vi "main program.vi"() -> ()   [LabVIEW 2015]
uses:
  <vilib>/rvi/interface/nirviReadWriteControl/nirviReadWriteControl.xnode
  <vilib>/rvi/interface/nirviMethod/nirviMethod.xnode
  <vilib>/rvi/interface/nirviCloseFPGA/nirviCloseFPGA.xnode
  <vilib>/FPGAPlugInAG/Dynamic/niLvFpga_Run_Dynamic.vi
  <vilib>/rvi/interface/Simulation/niFpgaSimulationCallBeginRW.vi
  <vilib>/rvi/errors/niLvFpgaAdjustHostInterfaceError.vi
  <vilib>/Platform/TimedLoop/XDataNode/XDataNode.xnode
  <vilib>/Platform/TimedLoop/XDataNode/nitl_modes.ctl
  <vilib>/Platform/TimedLoop/XDataNode/XDNodeRunTimeDep.lvlib
  <vilib>/Platform/TimedLoop/XDataNode/wakeup.ctl
  <vilib>/Platform/TimedLoop/XDataNode/timing_clust.ctl
  <vilib>/FPGAPlugInAG/Dynamic/niLvFpga_Close_Dynamic.vi
  <vilib>/vision/driver/NI_Vision_Acquisition_Software.lvlib
  <resource>/objmgr/imaqdx.rc
  <vilib>/addons/control/pid/NI_PID_pid.lvlib
  <vilib>/addons/control/pid/pid.llb/PID (DBL).vi
  <vilib>/addons/Fuzzy Logic/NI_Fuzzy_Logic_API.lvlib
  <vilib>/addons/Fuzzy Logic/FL Fuzzy Controller (MIMO).vi
  <vilib>/rvi/interface/nirviOpenFPGA/nirviOpenFPGA.xnode
  NiFpgaLv.dll
  <vilib>/Utility/error.llb/Error Cluster From Error Code.vi
  <vilib>/rvi/Arithmetic/AddSubMult/XNode/nirviSatArithmetic.xnode
  FPGA Bitfiles/FPGAv2_FPGATarget2_Assemble3_74ibksKrDUk.lvbitx
  Assemble.vi
  <vilib>/FPGAPlugInAG/myRIO-1900/niLvFpga_Open_myRIO-1900.vi
  <vilib>/rvi/interface/common/dynamic/niFpgaDynamicAddResources.vi
  <vilib>/userdefined/High Color/IMAQdx.ctl
panel:
  out "Battery percentage":dbl(slide) scale=0.0..100.0
  in  "file path":path=path "c:/captue.jpg"
  out "Distance":dbl
  in  "Capture pict.":bool
  out "video modes":string
  in  "video mode":u32=20
  out "?":T1(plugin-control)
  in  "webcam":T2="cam0"
  out "k.kanan":dbl
  out "k.kiri":dbl
  out "x-y 2":dbl
  out "x+y 2":dbl
  out "percp. 2":dbl
  out "w 2":dbl
  out "percp.":dbl
  out "w":dbl
  out "Velo":i32
  out "Acce":i32
  in  "interval 2":u32=1000
  out "Vel":i32
  out "Acc":i32
  in  "interval":u32=1000
  out "x-y":dbl
  out "x+y":dbl
  out "b":dbl
  out "a":dbl
  out "Velocity (Counts/Interval) 4":i32
  out "Velocity (Counts/Interval) 3":i32
  out "Velocity (Counts/Interval) 2":i32
  out "Velocity (Counts/Interval)":i32
  out "Acceleration (rps/s) 4":dbl
  out "Acceleration (rps/s) 3":dbl
  out "Acceleration (rps/s) 2":dbl
  out "Acceleration (rps/s)":dbl
  out "frame rate [fps]":dbl
  out "STOP Indicator":bool
  in  "Run/Stop":bool
  out "RC ch3":u32
  out "heading error":dbl
  out "target bearing":dbl
  out "target distance":dbl
  in  "y target":dbl
  in  "x target":dbl
  out "voltage":dbl
  out "var.RTH":dbl
  out "kec.kanan":dbl
  out "kec.kiri":dbl
  out "kecp.kanan":dbl
  out "kecp.kiri":dbl
  out "var.auto":dbl
  in  "Mode":bool
  in  "RTH":bool
  out "relay 4":bool
  out "relay 3":bool
  out "relay 2":bool
  out "relay1":bool
  out "bocor 2":bool
  out "Water_LVL2":dbl
  out "Water_LVL1":dbl
  out "bocor 1":bool
  out "Arus 4":dbl
  out "Arus 3":dbl
  out "Arus1":dbl
  out "Arus2":dbl
  out "En 8":bool
  out "En 7":bool
  out "En 6":bool
  out "En 5":bool
  out "En 4":bool
  out "En 3":bool
  out "En 2":bool
  out "En 1":bool
  out "Rpm 4":dbl
  out "Rpm 3":dbl
  out "Rpm 2":dbl
  out "Rpm 1":dbl
  out "To":dbl
  out "var. manual":dbl
  out "enc 4":i32
  out "enc 3":i32
  out "enc 2":i32
  out "enc 1":i32
  out "Time On4":dbl format="%.2f"
  out "Time On3":dbl format="%.2f"
  out "Time On2":dbl
  out "y position":dbl
  out "x position":dbl
  out "angle":dbl
  out "Toff":dbl
  out "Time On1":dbl
  out "ultrasonik4":sgl
  out "ultrasonik3":sgl
  out "ultrasonik2":sgl
  out "ultrasonik1":sgl
  out "RC ch2":u32
  out "RC ch1":u32
  out "US 4":u32
  out "US3":u32
  out "US2":u32
  out "US1":u32
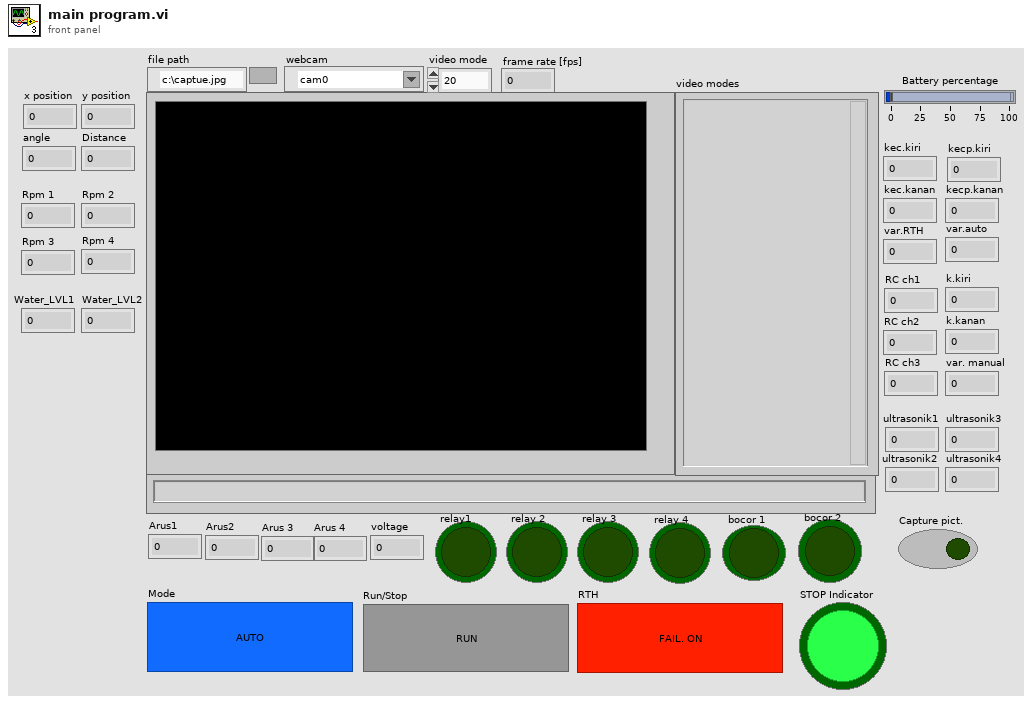
[diagram p1: front panel]
types:
  T1 = typedef "IMAQ Image.ctl" = refnum<image>
  T2 = typedef "IMAQdx.ctl" = refnum<k21>
  T3 = cluster{"Video Mode":u32, "Video Mode Name":string}[]
  T4 = typedef "XDNodeRunTimeDep.lvlib/timing_clust.ctl" = cluster{"Expected End [f-1]":u64, "Actual End [f-1]":u64, "Finished Late? [f-1]":bool, "Expected End [i-1]":u64, "Actual End [i-1]":u64, "Finished Late? [i-1]":bool, "Expected Start [i]":u64, "Actual Start [i]":u64, "Expected Start [f]":u64, "Actual Start [f]":u64, "Source Name":string, "Structure Name":string, "Period":i64, "Deadline":i64, "Offset":i64, "Start":i64, "Priority":i32, "Timeout":i32, "Mode":T5, "Wakeup Reason":T6, "Error":errorcluster, "Source Type":string, "Secondary Source Type":string, "Global End Time":u64, "Global Start Time":u64, "Frame Duration":u64, "Iteration Duration":u64, "Assigned CPU":i32, "I/O Scan Engine Mode":u32}
  T5 = typedef "XDNodeRunTimeDep.lvlib/nitl_modes.ctl" = enum32{"No Change", "Process missed periods, maintain original phase", "Discard missed periods, maintain original phase", "Process missed periods, ignore original phase", "Discard missed periods, ignore original phase"}
  T6 = typedef "XDNodeRunTimeDep.lvlib/wakeup.ctl" = enum32{"Normal", "Aborted", "Asynchronous wakeup", "Timing source error", "Timed loop error", "Timeout"}
  T7 = cluster{"proportional gain (Kc)":dbl, "integral time (Ti, min)":dbl, "derivative time (Td, min)":dbl}
  T8 = typedef "NI_Fuzzy_Logic_API.lvlib/FL System.ctl" = cluster{"input variables":T9[], "output variables":T9[], "rules":T12[], "defuzzification method":T18, "description":string, "user MF interpolating polynomials":T19[]}
  T9 = typedef "NI_Fuzzy_Logic_API.lvlib/FL Variable.ctl" = cluster{"name":string, "range":dbl[], "MFs":T10[]}
  T10 = typedef "NI_Fuzzy_Logic_API.lvlib/FL Membership Function.ctl" = cluster{"name":string, "shape":T11, "points":dbl[], "color":u32, "user-defined shape index":i32}
  T11 = typedef "NI_Fuzzy_Logic_API.lvlib/FL Membership Function Shape.ctl" = u16
  T12 = typedef "NI_Fuzzy_Logic_API.lvlib/FL Rule.ctl" = cluster{"antecedents":T13[], "antecedent connective":T15, "consequents":T16[], "consequent implication":T17, "degree of support":dbl}
  T13 = typedef "NI_Fuzzy_Logic_API.lvlib/FL Antecedent.ctl" = cluster{"Var Index":i32, "MF Index":i32, "Cond":T14}
  T14 = typedef "NI_Fuzzy_Logic_API.lvlib/FL Modifier.ctl" = u16
  T15 = typedef "NI_Fuzzy_Logic_API.lvlib/FL Antecedent Connective.ctl" = u16
  T16 = typedef "NI_Fuzzy_Logic_API.lvlib/FL Consequent.ctl" = cluster{"Var Index":i32, "MF Index":i32, "Cond":T14}
  T17 = typedef "NI_Fuzzy_Logic_API.lvlib/FL Consequent Implication.ctl" = u16
  T18 = typedef "NI_Fuzzy_Logic_API.lvlib/FL Defuzzification.ctl" = u16
  T19 = typedef "NI_Fuzzy_Logic_API.lvlib/FL Interpolating polynomials.ctl" = cluster{"X":dbl[], "Y":dbl[], "Y(x) coeff":dbl[][], "X(y) coeff":dbl[][], "Area(y) coeff":dbl[][], "coa_x(y) coeff":dbl[][]}
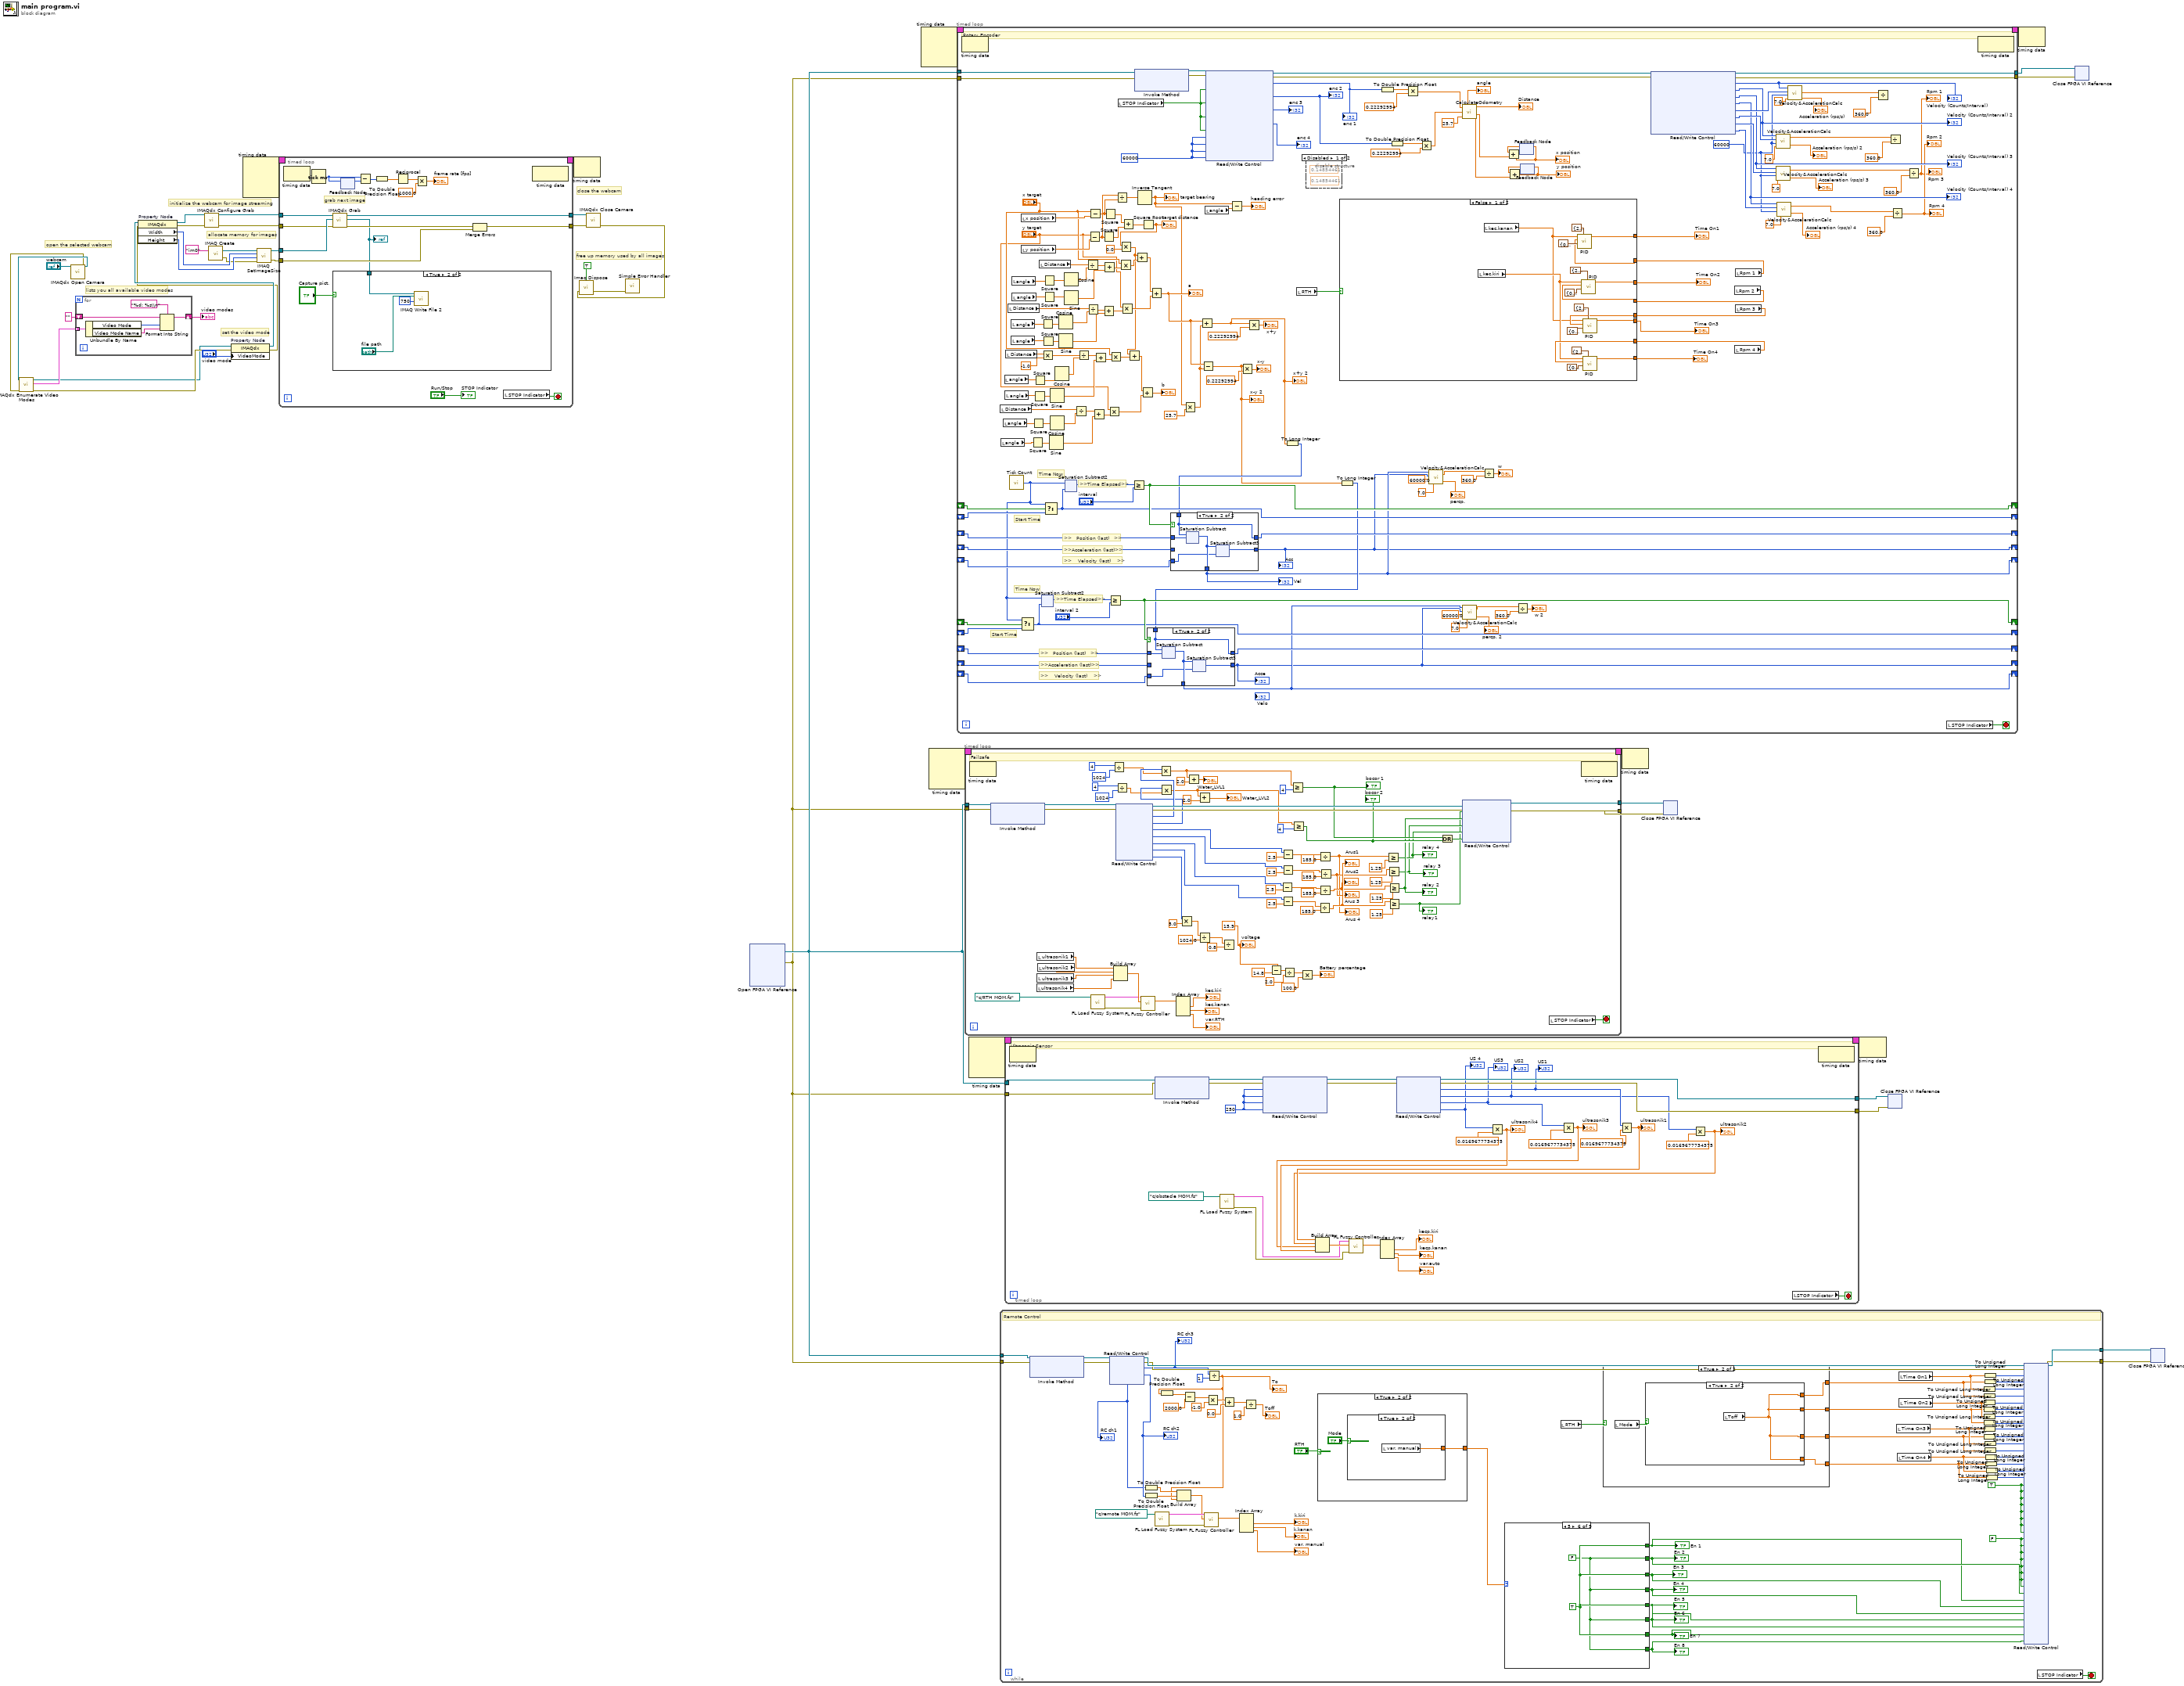
[diagram p0: block diagram]
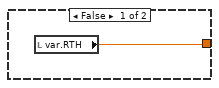
[diagram p3: hidden frame]
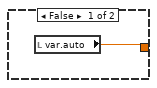
[diagram p4: hidden frame]
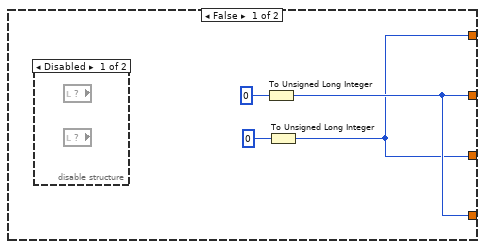
[diagram p5: hidden frame]
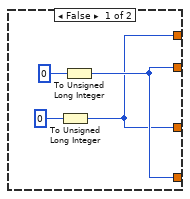
[diagram p7: hidden frame]
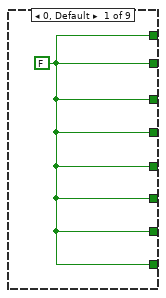
[diagram p8: hidden frame]
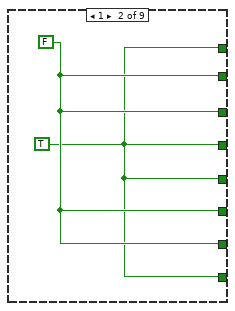
[diagram p9: hidden frame]
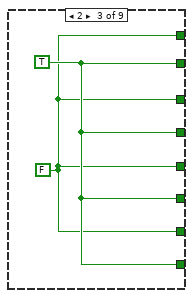
[diagram p10: hidden frame]
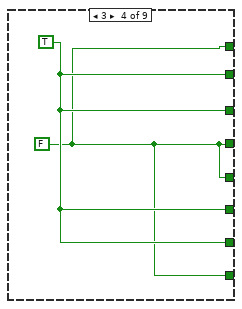
[diagram p11: hidden frame]
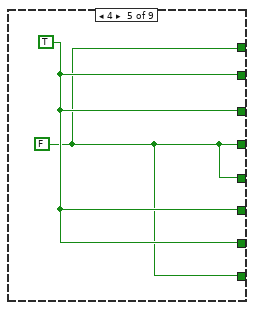
[diagram p12: hidden frame]
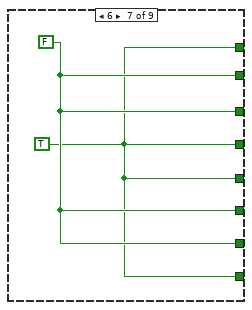
[diagram p13: hidden frame]
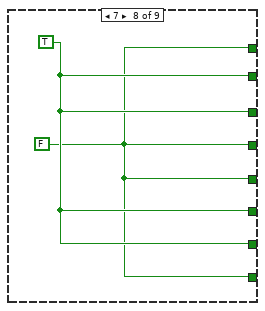
[diagram p14: hidden frame]
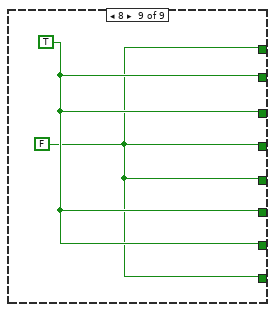
[diagram p15: hidden frame]
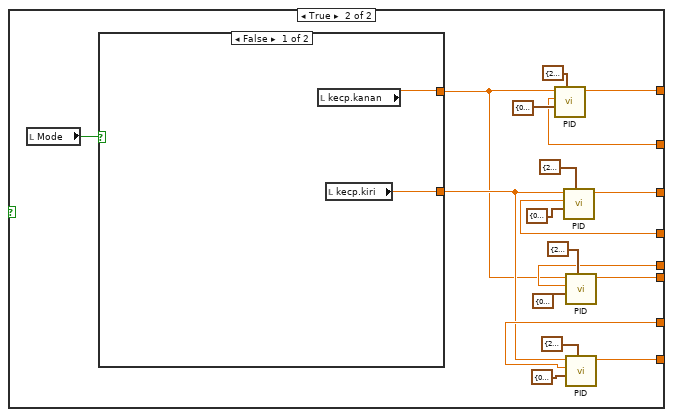
[diagram p19: hidden frame]
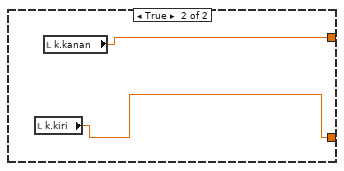
[diagram p20: hidden frame]
diagram:
  # "lists you all available video modes"
  # "close the webcam"
  # "open the selected webcam"
  # "set the video mode"
  # "allocate memory for images"
  # "initialize the webcam for image streaming"
  # "free up memory used by all images"
  n1 = call <vilib>:"IMAQdx Open Camera.vi"("Session In"="webcam") -> ("error out"=w5:errorcluster, "Session Out"=w6:T2)  [unwired: 2 in, 7 out]
  n2 = call <vilib>:"IMAQdx Enumerate Video Modes.vi"("error in"=w5, "Session In"=w6) -> ("error out"=w4:errorcluster, "Video Modes"=w9:T3, "Session Out"=w3:T2)  [unwired: 6 in, 1 out]
  n3 = for {
    tunnel: w9 -> [w51] mode=indexing
    shift-right: [w47] -> w8
    shift-left: "" -> [w46]
    n4 = Unbundle By Name(w51) -> ("Video Mode"=w49:u32, "Video Mode Name"=w48:string)
    n5 = Format Into String(format string="%d: %s\\n", initial string=w46, w49, w48) -> (resulting string=w47:string)  [unwired: 1 in, 1 out]
  }
  "video modes" <- w8
  n6 = call "IMAQ Create"("Image Name"="im0") -> ("New Image"=w19:T1, "error out"=w11:errorcluster)  [unwired: 3 in, 1 out]
  n7 = property on="Property Node" class="IMAQdx"(reference=w3, error in=w4, "VideoMode"="video mode") -> (reference out=w17:T2, error out=w14:errorcluster)
  n8 = property on="Property Node" class="IMAQdx"(reference=w17, error in=w14) -> (reference out=w16:T2, error out=w15:errorcluster, "Width"=w13:u32, "Height"=w12:u32)
  n9 = call <vilib>:"IMAQdx Configure Grab.vi"("error in"=w15, "Session In"=w16) -> ("error out"=w27:errorcluster, "Session Out"=w21:T2)  [unwired: 8 in]
  n10 = node-c288() -> (w2:T4)  [unwired: 4 in]
  n11 = call "IMAQ SetImageSize"("error in (no error)"=w11, "Y Resolution"=w12, "X Resolution"=w13, "Image"=w19) -> ("error out"=w10:errorcluster, "Image Out"=w18:T1)  [unwired: 1 in]
  n12 = timed-loop {
    tunnel: w18 -> [w69]
    tunnel: w27 -> [w67]
    tunnel: w21 -> [w68]
    tunnel: [w64] -> w24
    tunnel: [w65] -> w23
    tunnel: w10 -> [w54]
    timing: w2 -> [_]
    timing-out: [_] -> w1
    stop <- w62 stop-if-true
    # "grab next image"
    n13 = node-c288() -> ()  [unwired: 1 in, 1 out]
    n14 = Tick Count (ms)() -> (millisecond timer value=w61:u32)
    n15 = call <vilib>:"IMAQdx Grab.vi"("error in"=w67, "Image In"=w69, "Session In"=w68) -> ("error out"=w66:errorcluster, "Image Out"=w53:T1, "Session Out"=w65:T2)  [unwired: 5 in, 1 out]
    "?" <- w53
    n16 = case shown="True" "Capture pict." {
      tunnel: w53 -> [_ w72]
      frame False {
      }
      frame True {
        n17 = call-poly "IMAQ Write File 2"("Image Quality"=u32 750, "File Path"="file path", "Image"=w72) -> ()  [unwired: 7 in, 2 out]
      }
    }
    n18 = feedback #1() -> (w60:u32)  [unwired: 1 in]
    n19 = feedback-in #1(w61) -> ()
    n20 = Subtract(x=w61, y=w60) -> (x-y=w59:u32)
    n21 = To Double Precision Float(number=w59) -> (double precision float=w58:dbl)
    n22 = Reciprocal(x=w58) -> (1/x=w57:dbl)
    n23 = Multiply(x=w57, y=1000.0) -> (x*y=→"frame rate [fps]":dbl)
    n24 = Merge Errors(w66, w54) -> (w64:errorcluster)
    n25 = local read "STOP Indicator"() -> (w62:bool)
    n26 = node-c288() -> ()  [unwired: 1 in, 1 out]
    "STOP Indicator" <- "Run/Stop"
  }
  n27 = node-c288(w1) -> ()  [unwired: 1 out]
  n28 = call <vilib>:"IMAQdx Close Camera.vi"("error in"=w24, "Session In"=w23) -> ("error out"=w25:errorcluster)  [unwired: 9 out]
  n29 = call "Imaq Dispose"("All Images? (No)"=TRUE, "error in (no error)"=w25) -> ("error out"=w22:errorcluster)  [unwired: 4 in]
  n30 = call <vilib>:"Simple Error Handler.vi"("error in (no error)"=w22) -> ()  [unwired: 4 in, 5 out]
  n31 = xnode "Open FPGA VI Reference"() -> ("FPGA VI Reference Out"=w31:refnum<k20>, "error out"=w30:errorcluster)  [unwired: 2 in]
  n32 = node-c288() -> (w39:T4)  [unwired: 4 in]
  n33 = node-c288() -> (w35:T4)  [unwired: 4 in]
  n34 = timed-loop {
    timing: w39 -> [_]
    timing-out: [_] -> w38
    tunnel: w31 -> [w247]
    tunnel: w30 -> [w246]
    tunnel: [w240] -> w37
    tunnel: [w239] -> w36
    shift-right: [w133] -> _
    shift-left: _ -> [w138]
    shift-right: [w132] -> _
    shift-left: _ -> [w137]
    shift-right: [w131] -> _
    shift-left: _ -> [w136]
    shift-right: [w108] -> _
    shift-left: _ -> [w135]
    shift-right: [w109] -> _
    shift-left: _ -> [w134]
    shift-right: [w120] -> _
    shift-left: _ -> [w121]
    shift-right: [w119] -> _
    shift-left: _ -> [w122]
    shift-right: [w118] -> _
    shift-left: _ -> [w123]
    shift-right: [w100] -> _
    shift-left: _ -> [w124]
    shift-right: [w101] -> _
    shift-left: _ -> [w125]
    stop <- w245 stop-if-true
    w203 = u32 60000 ("Velocity Interval (uSec) 4")
    w204 = u32 60000 ("Velocity Interval (uSec) 4")
    # ">>Acceleration (last)>>"
    # "Start Time"
    # ">>    Velocity (last)    >>"
    # ">>   Position (last)   >>"
    # "Time Now"
    # ">>Time Elapsed>>"
    # ">>Acceleration (last)>>"
    # "Start Time"
    # ">>    Velocity (last)    >>"
    # ">>   Position (last)   >>"
    # "Time Now"
    # ">>Time Elapsed>>"
    # "Rotary Encoder"
    n35 = node-c288() -> ()  [unwired: 1 in, 1 out]
    n36 = local read "Distance"() -> (w88:dbl)
    n37 = local read "angle"() -> (w156:dbl)
    n38 = local read "angle"() -> (w161:dbl)
    n39 = local read "angle"() -> (w170:dbl)
    n40 = local read "angle"() -> (w166:dbl)
    n41 = local read "Distance"() -> (w89:dbl)
    n42 = local read "Distance"() -> (w90:dbl)
    n43 = call "Tick Count"() -> ("Tick Count(uSec)"=w126:u32)
    n44 = local read "angle"() -> (w187:dbl)
    n45 = local read "angle"() -> (w183:dbl)
    n46 = local read "angle"() -> (w194:dbl)
    n47 = local read "angle"() -> (w191:dbl)
    n48 = Select(t=w126, s=w121, f=w122) -> (s? t:f=w119:u32)
    n49 = local read "x position"() -> (w229:dbl)
    n50 = local read "y position"() -> (w228:dbl)
    n51 = Square(x=w156) -> (x^2=w157:dbl)
    n52 = Square(x=w161) -> (x^2=w160:dbl)
    n53 = Square(x=w166) -> (x^2=w167:dbl)
    n54 = Square(x=w170) -> (x^2=w171:dbl)
    n55 = local read "Distance"() -> (w91:dbl)
    n56 = Square(x=w187) -> (x^2=w186:dbl)
    n57 = Multiply(x=w89, y=-1.0) -> (x*y=w172:dbl)
    n58 = Square(x=w183) -> (x^2=w182:dbl)
    n59 = xnode ("Saturation Subtract2")("x"=w126, "y"=w119) -> ("x-y"=w127:u32)
    n60 = Square(x=w194) -> (x^2=w193:dbl)
    n61 = Square(x=w191) -> (x^2=w190:dbl)
    n62 = Select(t=w126, s=w138, f=w137) -> (s? t:f=w132:u32)
    n63 = Sine(x=w157) -> (sin(x)=w158:dbl)
    n64 = Cosine(x=w160) -> (cos(x)=w159:dbl)
    n65 = Sine(x=w167) -> (sin(x)=w165:dbl)
    n66 = Cosine(x=w171) -> (cos(x)=w169:dbl)
    n67 = Cosine(x=w186) -> (cos(x)=w185:dbl)
    n68 = Sine(x=w182) -> (sin(x)=w181:dbl)
    n69 = Cosine(x=w193) -> (cos(x)=w192:dbl)
    n70 = Sine(x=w190) -> (sin(x)=w189:dbl)
    n71 = xnode ("Saturation Subtract2")("x"=w126, "y"=w132) -> ("x-y"=w139:u32)
    n72 = Divide(x=w88, y=w159) -> (x/y=w162:dbl)
    n73 = Divide(x=w172, y=w169) -> (x/y=w168:dbl)
    n74 = Divide(x=w91, y=w192) -> (x/y=w188:dbl)
    n75 = Divide(x=w90, y=w185) -> (x/y=w184:dbl)
    n76 = Subtract(x="y target", y=w228) -> (x-y=w227:dbl)
    n77 = Subtract(x="x target", y=w229) -> (x-y=w226:dbl)
    n78 = Add(x=w162, y=w158) -> (x+y=w155:dbl)
    n79 = Add(x=w168, y=w165) -> (x+y=w164:dbl)
    n80 = Square(x=w227) -> (x^2=w231:dbl)
    n81 = Add(x=w184, y=w181) -> (x+y=w179:dbl)
    n82 = Add(x=w188, y=w189) -> (x+y=w180:dbl)
    n83 = Square(x=w226) -> (x^2=w232:dbl)
    n84 = Multiply(x="y target", y=w155) -> (x*y=w150:dbl)
    n85 = Greater Or Equal?(x=w127, y="interval 2") -> (x >= y?=w120:bool)
    n86 = Multiply(x="x target", y=w164) -> (x*y=w153:dbl)
    n87 = Divide(x=w227, y=w226) -> (x/y=w225:dbl)
    n88 = local read "STOP Indicator"() -> (w96:bool)
    n89 = Multiply(x="x target", y=w180) -> (x*y=w176:dbl)
    n90 = Multiply(x="y target", y=w179) -> (x*y=w174:dbl)
    n91 = Add(x=w232, y=w231) -> (x+y=w230:dbl)
    n92 = Greater Or Equal?(x=w139, y="interval") -> (x >= y?=w133:bool)
    n93 = xnode "Invoke Method"("FPGA VI Reference In"=w247, "error in"=w246) -> ("FPGA VI Reference Out"=w249:refnum<k20>, "error out"=w248:errorcluster)  [unwired: 1 in]
    n94 = Inverse Tangent(1:w225) -> (0:w145:dbl)
    "target bearing" <- w145
    n95 = Square Root(x=w230) -> (sqrt(x)=w177:dbl)
    "target distance" <- w177
    n96 = Multiply(x=w177, y=0.0) -> (x*y=w152:dbl)
    n97 = Add(x=w152, y=w153) -> (x+y=w151:dbl)
    n98 = Add(x=w152, y=w176) -> (x+y=w175:dbl)
    n99 = Add(x=w151, y=w150) -> (x+y=→"b":dbl)
    n100 = Add(x=w175, y=w174) -> (x+y=w147:dbl)
    "a" <- w147
    n101 = Multiply(x=w145, y=25.7) -> (x*y=w146:dbl)
    n102 = Add(x=w147, y=w146) -> (x+y=w130:dbl)
    "x+y 2" <- w130
    n103 = Subtract(x=w147, y=w146) -> (x-y=w116:dbl)
    "x-y 2" <- w116
    n104 = local read "angle"() -> (w223:dbl)
    n105 = xnode "Read/Write Control"("FPGA VI Reference In"=w249, "error in"=w248, "Position Reset"=w96, "Position Reset 2"=w96, "Position Reset 3"=w96, "Position Reset 4"=w96, "Velocity Interval (uSec)"=w204, "Velocity Interval (uSec) 2"=w204, "Velocity Interval (uSec) 3"=w204, "Velocity Interval (uSec) 4"=w204) -> ("FPGA VI Reference Out"=w238:refnum<k20>, "error out"=w237:errorcluster, "Position 1"=w81:i32, "Position 2"=w80:i32, "Position 3"=→"enc 3":i32, "Position 4"=→"enc 4":i32)
    "enc 1" <- w81
    "enc 2" <- w80
    n106 = Subtract(x=w145, y=w223) -> (x-y=→"heading error":dbl)
    n107 = Multiply(x=w116, y=0.22292994) -> (x*y=→"x-y":dbl)
    n108 = Multiply(x=w130, y=0.22292994) -> (x*y=→"x+y":dbl)
    n109 = To Long Integer(number=w130) -> (32bit integer=w129:i32)
    n110 = case shown="True" w133 {
      tunnel: w129 -> [_ w317]
      tunnel: w136 -> [w314 w321]
      tunnel: [w316 w320] -> w109
      tunnel: w134 -> [w316 w319]
      tunnel: [w315 w318] -> w108
      tunnel: w135 -> [w315 _]
      tunnel: [w314 w317] -> w131
      frame False {
      }
      frame True {
        n111 = xnode ("Saturation Subtract")("x"=w317, "y"=w321) -> ("x-y"=w320:i32)
        n112 = xnode ("Saturation Subtract3")("x"=w320, "y"=w319) -> ("x-y"=w318:i32)
      }
    }
    "Acc" <- w108
    "Vel" <- w109
    n113 = local read "RTH"() -> (w233:bool)
    n114 = disable-structure shown="Disabled" {
      frame Disabled {
        (unwired) 0.14854461 ("y")
        (unwired) 0.14854461 ("y")
      }
      frame Enabled {
      }
    }
    n115 = To Long Integer(number=w116) -> (32bit integer=w117:i32)
    n116 = case shown="True" w120 {
      tunnel: w117 -> [_ w263]
      tunnel: w123 -> [w260 w267]
      tunnel: [w262 w266] -> w101
      tunnel: w125 -> [w262 w265]
      tunnel: [w261 w264] -> w100
      tunnel: w124 -> [w261 _]
      tunnel: [w260 w263] -> w118
      frame False {
      }
      frame True {
        n117 = xnode ("Saturation Subtract")("x"=w263, "y"=w267) -> ("x-y"=w266:i32)
        n118 = xnode ("Saturation Subtract3")("x"=w266, "y"=w265) -> ("x-y"=w264:i32)
      }
    }
    "Acce" <- w100
    n119 = To Double Precision Float(number=w81) -> (double precision float=w244:dbl)
    n120 = To Double Precision Float(number=w80) -> (double precision float=w243:dbl)
    n121 = Multiply(x=w244, y=0.22292994) -> (x*y=w95:dbl)
    n122 = Multiply(x=w243, y=0.22292994) -> (x*y=w94:dbl)
    n123 = call "Velocity&AccelerationCalc.vi"("Pulses/Revolution"=7.0 ("y"), "Fixed Time \nInterval (uSec)"=60000.0 ("Fixed Time \nInterval (uSec)"), "Acceleration (Counts/Interval)"=w108, "Velocity (Counts/Interval)"=w109) -> ("Acceleration (rps/s)"=→"percp.":dbl, "Velocity (RPM)"=w112:dbl)
    n124 = call "CalculateOdometry.vi"("Left Wheel Distance"=w95, "Right Wheel Distance"=w94, "Wheel Base"=25.7) -> ("Distance"=→"Distance":dbl, "X"=w83:dbl, "Y"=w82:dbl, "Heading"=→"angle":dbl)  [unwired: 1 out]
    n125 = call "Velocity&AccelerationCalc.vi"("Pulses/Revolution"=7.0 ("y"), "Fixed Time \nInterval (uSec)"=60000.0 ("Fixed Time \nInterval (uSec)"), "Acceleration (Counts/Interval)"=w100, "Velocity (Counts/Interval)"=w101) -> ("Acceleration (rps/s)"=→"percp. 2":dbl, "Velocity (RPM)"=w104:dbl)
    n126 = Divide(x=w112, y=360.0) -> (x/y=→"w":dbl)
    n127 = Divide(x=w104, y=360.0) -> (x/y=→"w 2":dbl)
    n128 = feedback #2() -> (w86:dbl)  [unwired: 1 in]
    n129 = Add(x=w86, y=w83) -> (x+y=w85:dbl)
    "x position" <- w85
    n130 = feedback-in #2(w85) -> ()
    n131 = feedback #3() -> (w87:dbl)  [unwired: 1 in]
    n132 = Add(x=w87, y=w82) -> (x+y=w84:dbl)
    "y position" <- w84
    n133 = feedback-in #3(w84) -> ()
    n134 = xnode "Read/Write Control"("FPGA VI Reference In"=w238, "error in"=w237) -> ("FPGA VI Reference Out"=w240:refnum<k20>, "error out"=w239:errorcluster, "Velocity (Counts/Interval)"=w98:i32, "Velocity (Counts/Interval) 2"=w214:i32, "Velocity (Counts/Interval) 3"=w213:i32, "Velocity (Counts/Interval) 4"=w212:i32, "Acceleration (Counts/Interval)"=w222:i32, "Acceleration (Counts/Interval) 2"=w220:i32, "Acceleration (Counts/Interval) 3"=w219:i32, "Acceleration (Counts/Interval) 4"=w218:i32)
    "Velocity (Counts/Interval)" <- w98
    "Velocity (Counts/Interval) 2" <- w214
    "Velocity (Counts/Interval) 3" <- w213
    "Velocity (Counts/Interval) 4" <- w212
    n135 = local read "Rpm 2"() -> (w205:dbl)
    n136 = local read "Rpm 4"() -> (w207:dbl)
    n137 = local read "Rpm 1"() -> (w97:dbl)
    n138 = local read "Rpm 3"() -> (w206:dbl)
    n139 = case shown="False" w233 {
      tunnel: w97 -> [w366 w391]
      tunnel: [w367 w390] -> w99
      tunnel: [w365 w387] -> w236
      tunnel: w205 -> [w364 w386]
      tunnel: w206 -> [w363 w383]
      tunnel: [w362 w382] -> w235
      tunnel: [w360 w379] -> w234
      tunnel: w207 -> [w361 w378]
      frame False {
        n140 = local read "kec.kiri"() -> (w359:dbl)
        n141 = local read "kec.kanan"() -> (w358:dbl)
        n142 = call-poly <vilib>:"PID.vi"("output range"=cluster{"output high":dbl, "output low":dbl} {"output high"=2000.0, "output low"=0.0}, "PID gains"=T7 {"proportional gain (Kc)"=0.3, "integral time (Ti, min)"=0.75, "derivative time (Td, min)"=0.1875}, "process variable"=w366, "setpoint"=w358) -> ("output"=w367:dbl)  [unwired: 6 in, 1 out]
        n143 = call-poly <vilib>:"PID.vi"("output range"=cluster{"output high":dbl, "output low":dbl} {"output high"=2000.0, "output low"=0.0}, "PID gains"=T7 {"proportional gain (Kc)"=0.3, "integral time (Ti, min)"=0.75, "derivative time (Td, min)"=0.1875}, "process variable"=w364, "setpoint"=w359) -> ("output"=w365:dbl)  [unwired: 6 in, 1 out]
        n144 = call-poly <vilib>:"PID.vi"("output range"=cluster{"output high":dbl, "output low":dbl} {"output high"=2000.0, "output low"=0.0}, "PID gains"=T7 {"proportional gain (Kc)"=0.3, "integral time (Ti, min)"=0.75, "derivative time (Td, min)"=0.1875}, "process variable"=w363, "setpoint"=w358) -> ("output"=w362:dbl)  [unwired: 6 in, 1 out]
        n145 = call-poly <vilib>:"PID.vi"("output range"=cluster{"output high":dbl, "output low":dbl} {"output high"=2000.0, "output low"=0.0}, "PID gains"=T7 {"proportional gain (Kc)"=0.3, "integral time (Ti, min)"=0.75, "derivative time (Td, min)"=0.1875}, "process variable"=w361, "setpoint"=w359) -> ("output"=w360:dbl)  [unwired: 6 in, 1 out]
      }
      frame True {
        n146 = local read "Mode"() -> (w394:bool)
        n147 = case shown="False" w394 {
          tunnel: [w395 w397] -> w377
          tunnel: [w396 w398] -> w376
          frame False {
            n148 = local read "kecp.kanan"() -> (w396:dbl)
            n149 = local read "kecp.kiri"() -> (w395:dbl)
          }
          frame True {
            n150 = local read "k.kiri"() -> (w397:dbl)
            n151 = local read "k.kanan"() -> (w398:dbl)
          }
        }
        n152 = call-poly <vilib>:"PID.vi"("output range"=cluster{"output high":dbl, "output low":dbl} {"output high"=2000.0, "output low"=0.0}, "PID gains"=T7 {"proportional gain (Kc)"=0.3, "integral time (Ti, min)"=0.75, "derivative time (Td, min)"=0.1875}, "process variable"=w391, "setpoint"=w376) -> ("output"=w390:dbl)  [unwired: 6 in, 1 out]
        n153 = call-poly <vilib>:"PID.vi"("output range"=cluster{"output high":dbl, "output low":dbl} {"output high"=2000.0, "output low"=0.0}, "PID gains"=T7 {"proportional gain (Kc)"=0.3, "integral time (Ti, min)"=0.75, "derivative time (Td, min)"=0.1875}, "process variable"=w386, "setpoint"=w377) -> ("output"=w387:dbl)  [unwired: 6 in, 1 out]
        n154 = call-poly <vilib>:"PID.vi"("output range"=cluster{"output high":dbl, "output low":dbl} {"output high"=2000.0, "output low"=0.0}, "PID gains"=T7 {"proportional gain (Kc)"=0.3, "integral time (Ti, min)"=0.75, "derivative time (Td, min)"=0.1875}, "process variable"=w383, "setpoint"=w376) -> ("output"=w382:dbl)  [unwired: 6 in, 1 out]
        n155 = call-poly <vilib>:"PID.vi"("output range"=cluster{"output high":dbl, "output low":dbl} {"output high"=2000.0, "output low"=0.0}, "PID gains"=T7 {"proportional gain (Kc)"=0.3, "integral time (Ti, min)"=0.75, "derivative time (Td, min)"=0.1875}, "process variable"=w378, "setpoint"=w377) -> ("output"=w379:dbl)  [unwired: 6 in, 1 out]
      }
    }
    "Time On1" <- w99
    "Time On2" <- w236
    "Time On3" <- w235
    "Time On4" <- w234
    n156 = call "Velocity&AccelerationCalc.vi"("Pulses/Revolution"=7.0 ("y"), "Fixed Time \nInterval (uSec)"=w203, "Acceleration (Counts/Interval)"=w220, "Velocity (Counts/Interval)"=w214) -> ("Acceleration (rps/s)"=→"Acceleration (rps/s) 2":dbl, "Velocity (RPM)"=w199:dbl)
    n157 = call "Velocity&AccelerationCalc.vi"("Pulses/Revolution"=7.0 ("y"), "Fixed Time \nInterval (uSec)"=w203, "Acceleration (Counts/Interval)"=w219, "Velocity (Counts/Interval)"=w213) -> ("Acceleration (rps/s)"=→"Acceleration (rps/s) 3":dbl, "Velocity (RPM)"=w197:dbl)
    n158 = call "Velocity&AccelerationCalc.vi"("Pulses/Revolution"=7.0 ("y"), "Fixed Time \nInterval (uSec)"=w203, "Acceleration (Counts/Interval)"=w218, "Velocity (Counts/Interval)"=w212) -> ("Acceleration (rps/s)"=→"Acceleration (rps/s) 4":dbl, "Velocity (RPM)"=w195:dbl)
    n159 = call "Velocity&AccelerationCalc.vi"("Pulses/Revolution"=7.0 ("y"), "Fixed Time \nInterval (uSec)"=w203, "Acceleration (Counts/Interval)"=w222, "Velocity (Counts/Interval)"=w98) -> ("Acceleration (rps/s)"=→"Acceleration (rps/s)":dbl, "Velocity (RPM)"=w202:dbl)
    n160 = Divide(x=w202, y=360.0) -> ()  [unwired: 1 out]
    n161 = Divide(x=w199, y=360.0) -> ()  [unwired: 1 out]
    n162 = Divide(x=w195, y=360.0) -> (x/y=→"Rpm 2" →"Rpm 4":dbl)
    n163 = Divide(x=w197, y=360.0) -> (x/y=→"Rpm 1" →"Rpm 3":dbl)
    n164 = local read "STOP Indicator"() -> (w245:bool)
    n165 = node-c288() -> ()  [unwired: 1 in, 1 out]
  }
  n166 = timed-loop {
    timing: w35 -> [_]
    timing-out: [_] -> w34
    tunnel: w31 -> [w481]
    tunnel: w30 -> [w480]
    tunnel: [w475] -> w33
    tunnel: [w474] -> w32
    stop <- w473 stop-if-true
    w405 = 15.9 ("voltage")
    # "Failsafe"
    n167 = node-c288() -> ()  [unwired: 1 in, 1 out]
    n168 = xnode "Invoke Method"("FPGA VI Reference In"=w481, "error in"=w480) -> ("FPGA VI Reference Out"=w479:refnum<k20>, "error out"=w478:errorcluster)  [unwired: 1 in]
    n169 = local read "ultrasonik4"() -> (w462:sgl)
    n170 = local read "ultrasonik1"() -> (w459:sgl)
    n171 = local read "ultrasonik3"() -> (w461:sgl)
    n172 = local read "ultrasonik2"() -> (w460:sgl)
    n173 = call <vilib>:"FL Load Fuzzy System.vi"("file path"=path "c:/RTH MOM.fs") -> ("error out"=w457:errorcluster, "fuzzy system out"=w456:T8)  [unwired: 1 in, 8 out]
    n174 = Divide(x=u16 4 ("y"), y=u16 1024) -> (x/y=w444:dbl)
    n175 = Build Array(w459, w460, w461, w462) -> (w458:sgl[])
    n176 = Divide(x=u16 4 ("y"), y=u16 1024) -> (x/y=w445:dbl)
    n177 = xnode "Read/Write Control"("FPGA VI Reference In"=w479, "error in"=w478) -> ("FPGA VI Reference Out"=w477:refnum<k20>, "error out"=w476:errorcluster, "Water_LVL1"=w451:u16, "Water_LVL2"=w450:u16, "ACS712(1)"=w428:u16, "ACS712(2)"=w427:u16, "ACS712(3)"=w426:u16, "ACS712(4)"=w425:u16, "V sensor"=w465:u16)
    n178 = call-poly <vilib>:"FL Fuzzy Controller.vi"("error in (no error)"=w457, "input values"=w458, "fuzzy system in"=w456) -> ("output values"=w455:dbl[])  [unwired: 8 out]
    n179 = Multiply(x=w451, y=w444) -> (x*y=w424:dbl)
    n180 = Multiply(x=w450, y=w445) -> (x*y=w423:dbl)
    n181 = Index Array(array=w455) -> (element #1=→"kec.kiri":dbl, element #2=→"kec.kanan":dbl, element #3=→"var.RTH":dbl)  [unwired: 3 in]
    n182 = Multiply(x=w465, y=5.0) -> (x*y=w464:dbl)
    n183 = Add(x=w424, y=2.0) -> (x+y=→"Water_LVL1":dbl)
    n184 = Add(x=w423, y=2.0) -> (x+y=→"Water_LVL2":dbl)
    n185 = Divide(x=w464, y=1024.0) -> (x/y=w452:dbl)
    n186 = Divide(x=w452, y=0.8) -> ()  [unwired: 1 out]
    n187 = Subtract(x=w405, y=14.8) -> (x-y=w422:dbl)
    n188 = Subtract(x=w426, y=2.5) -> (x-y=w431:dbl)
    n189 = Subtract(x=w428, y=2.5) -> (x-y=w435:dbl)
    n190 = Subtract(x=w427, y=2.5) -> (x-y=w433:dbl)
    n191 = Subtract(x=w425, y=2.5) -> (x-y=w429:dbl)
    n192 = Divide(x=w422, y=2.0) -> (x/y=w420:dbl)
    n193 = Greater Or Equal?(x=w424, y=u16 4) -> (x >= y?=w413:bool)
    "bocor 1" <- w413
    n194 = Greater Or Equal?(x=w423, y=u16 4) -> (x >= y?=w412:bool)
    "bocor 2" <- w412
    n195 = Multiply(x=w420, y=100.0) -> (x*y=→"Battery percentage":dbl)
    n196 = Divide(x=w429, y=185.0) -> (x/y=w404:dbl)
    "Arus1" <- w404
    n197 = Divide(x=w435, y=185.0) -> (x/y=w401:dbl)
    "Arus 4" <- w401
    n198 = Divide(x=w431, y=185.0) -> (x/y=w403:dbl)
    "Arus2" <- w403
    n199 = Divide(x=w433, y=185.0) -> (x/y=w402:dbl)
    "Arus 3" <- w402
    n200 = Greater Or Equal?(x=w401, y=1.25) -> (x >= y?=w410:bool)
    "relay 4" <- w410
    n201 = Greater Or Equal?(x=w402, y=1.25) -> (x >= y?=w407:bool)
    "relay 3" <- w407
    n202 = Greater Or Equal?(x=w403, y=1.25) -> (x >= y?=w411:bool)
    "relay 2" <- w411
    n203 = Greater Or Equal?(x=w404, y=1.25) -> (x >= y?=w406:bool)
    "relay1" <- w406
    n204 = Or(x=w413, y=w412) -> (x .or. y?=w408:bool)
    n205 = xnode "Read/Write Control"("FPGA VI Reference In"=w477, "error in"=w476, "Relay Motor 1"=w406, "Relay motor 2"=w411, "Relay motor 3"=w407, "Relay motor 4"=w410, "Relay kebocoran"=w408) -> ("FPGA VI Reference Out"=w475:refnum<k20>, "error out"=w474:errorcluster)
    n206 = local read "STOP Indicator"() -> (w473:bool)
    n207 = node-c288() -> ()  [unwired: 1 in, 1 out]
    "voltage" <- w405
  }
  n208 = node-c288() -> (w43:T4)  [unwired: 4 in]
  n209 = while {
    tunnel: [w542] -> w45
    tunnel: [w540] -> w44
    tunnel: w31 -> [w552]
    tunnel: w30 -> [w551]
    stop <- w553 stop-if-true
    w513 = FALSE ("E2O")
    w514 = TRUE ("E2O")
    # "Remote Control"
    n210 = xnode "Invoke Method"("FPGA VI Reference In"=w552, "error in"=w551) -> ("FPGA VI Reference Out"=w550:refnum<k20>, "error out"=w549:errorcluster)  [unwired: 1 in]
    n211 = xnode "Read/Write Control"("FPGA VI Reference In"=w550, "error in"=w549) -> ("FPGA VI Reference Out"=w541:refnum<k20>, "error out"=w539:errorcluster, "Channel 3"=w494:u32, "Channel) 2"=w493:u32, "Channel 1"=w492:u32)
    "RC ch1" <- w492
    "RC ch2" <- w493
    "RC ch3" <- w494
    n212 = To Double Precision Float(number=w492) -> (double precision float=w502:dbl)
    n213 = To Double Precision Float(number=w493) -> (double precision float=w503:dbl)
    n214 = call <vilib>:"FL Load Fuzzy System.vi"("file path"=path "c:/remote MOM.fs") -> ("error out"=w506:errorcluster, "fuzzy system out"=w505:T8)  [unwired: 1 in, 8 out]
    n215 = Divide(x=w494, y=u32 1) -> (x/y=w495:dbl)
    "To" <- w495
    n216 = To Double Precision Float(number=w495) -> (double precision float=w543:dbl)
    n217 = Build Array(w502, w503, w495) -> (w501:dbl[])
    n218 = Subtract(x=w543, y=sgl 2000.0) -> (x-y=w548:dbl)
    n219 = call-poly <vilib>:"FL Fuzzy Controller.vi"("error in (no error)"=w506, "input values"=w501, "fuzzy system in"=w505) -> ("output values"=w504:dbl[])  [unwired: 8 out]
    n220 = Multiply(x=w548, y=sgl -1.0) -> (x*y=w547:dbl)
    n221 = Add(x=w547, y=sgl 0.0 ("-y")) -> (x+y=w532:dbl)
    n222 = Index Array(array=w504) -> (element #1=→"k.kiri":dbl, element #2=→"k.kanan":dbl, element #3=→"var. manual":dbl)  [unwired: 3 in]
    n223 = Divide(x=w532, y=1.0) -> (x/y=→"Toff":dbl)
    n224 = case shown="True" "RTH" {
      tunnel: [w554 w555] -> w507
      frame False {
        n225 = local read "var.RTH"() -> (w554:dbl)
      }
      frame True {
        n226 = case shown="True" "Mode" {
          tunnel: [w557 w558] -> w555
          frame False {
            n227 = local read "var.auto"() -> (w557:dbl)
          }
          frame True {
            n228 = local read "var. manual"() -> (w558:dbl)
          }
        }
      }
    }
    n229 = case shown="5" w507 {
      tunnel: [w573 w574 w576 w578 w580 w583 w584 w586 w588] -> w490
      tunnel: [w573 w575 w577 w579 w581 w582 w585 w587 w589] -> w491
      tunnel: [w573 w575 w576 w579 w581 w583 w585 w587 w589] -> w489
      tunnel: [w573 w574 w577 w578 w580 w582 w584 w586 w588] -> w488
      tunnel: [w573 w574 w576 w578 w580 w583 w584 w586 w588] -> w511
      tunnel: [w573 w575 w577 w579 w581 w582 w585 w587 w589] -> w512
      tunnel: [w573 w575 w576 w579 w581 w583 w585 w587 w589] -> w510
      tunnel: [w573 w574 w577 w578 w580 w582 w584 w586 w588] -> w509
      frame 0, Default {
        w573 = FALSE ("En")
      }
      frame 1 {
        w574 = TRUE ("En")
        w575 = FALSE ("En")
      }
      frame 2 {
        w576 = FALSE ("En")
        w577 = TRUE ("En")
      }
      frame 3 {
        w578 = FALSE ("En")
        w579 = TRUE ("En")
      }
      frame 4 {
        w580 = FALSE ("En")
        w581 = TRUE ("En")
      }
      frame 5 {
        w583 = TRUE ("En")
        w582 = FALSE ("En")
      }
      frame 6 {
        w584 = TRUE ("En")
        w585 = FALSE ("En")
      }
      frame 7 {
        w586 = FALSE ("En")
        w587 = TRUE ("En")
      }
      frame 8 {
        w588 = FALSE ("En")
        w589 = TRUE ("En")
      }
    }
    "En 1" <- w490
    "En 2" <- w491
    "En 3" <- w489
    "En 4" <- w488
    "En 5" <- w511
    "En 6" <- w512
    "En 7" <- w510
    "En 8" <- w509
    n230 = local read "RTH"() -> (w534:bool)
    n231 = case shown="True" w534 {
      tunnel: [w561 w566] -> w485
      tunnel: [w562 w565] -> w484
      tunnel: [w561 w564] -> w517
      tunnel: [w562 w563] -> w515
      frame False {
        n232 = disable-structure shown="Disabled" {
          frame Disabled {
            n233 = local read item#-1() -> ()  [unwired: 1 out]
            n234 = local read item#-1() -> ()  [unwired: 1 out]
          }
          frame Enabled {
          }
        }
        n235 = To Unsigned Long Integer(number=u32 0) -> (unsigned 32bit integer=w562:u32)
        n236 = To Unsigned Long Integer(number=u32 0) -> (unsigned 32bit integer=w561:u32)
      }
      frame True {
        n237 = local read "Mode"() -> (w567:bool)
        n238 = case shown="True" w567 {
          tunnel: [w570 w572] -> w566
          tunnel: [w571 w572] -> w565
          tunnel: [w570 w572] -> w564
          tunnel: [w571 w572] -> w563
          frame False {
            n239 = To Unsigned Long Integer(number=u32 0) -> (unsigned 32bit integer=w570:u32)
            n240 = To Unsigned Long Integer(number=u32 0) -> (unsigned 32bit integer=w571:u32)
          }
          frame True {
            n241 = local read "Toff"() -> (w572:dbl)
          }
        }
      }
    }
    n242 = local read "Time On3"() -> (w518:dbl)
    n243 = local read "Time On4"() -> (w516:dbl)
    n244 = local read "Time On1"() -> (w487:dbl)
    n245 = local read "Time On2"() -> (w486:dbl)
    n246 = To Unsigned Long Integer(number=w487) -> (unsigned 32bit integer=w537:u32)
    n247 = To Unsigned Long Integer(number=w484) -> (unsigned 32bit integer=w528:u32)
    n248 = To Unsigned Long Integer(number=w486) -> (unsigned 32bit integer=w535:u32)
    n249 = To Unsigned Long Integer(number=w484) -> (unsigned 32bit integer=w527:u32)
    n250 = To Unsigned Long Integer(number=w518) -> (unsigned 32bit integer=w526:u32)
    n251 = To Unsigned Long Integer(number=w485) -> (unsigned 32bit integer=w529:u32)
    n252 = To Unsigned Long Integer(number=w486) -> (unsigned 32bit integer=w536:u32)
    n253 = To Unsigned Long Integer(number=w517) -> (unsigned 32bit integer=w525:u32)
    n254 = To Unsigned Long Integer(number=w487) -> (unsigned 32bit integer=w538:u32)
    n255 = To Unsigned Long Integer(number=w485) -> (unsigned 32bit integer=w530:u32)
    n256 = To Unsigned Long Integer(number=w518) -> (unsigned 32bit integer=w524:u32)
    n257 = To Unsigned Long Integer(number=w517) -> (unsigned 32bit integer=w523:u32)
    n258 = To Unsigned Long Integer(number=w516) -> (unsigned 32bit integer=w522:u32)
    n259 = To Unsigned Long Integer(number=w515) -> (unsigned 32bit integer=w521:u32)
    n260 = To Unsigned Long Integer(number=w516) -> (unsigned 32bit integer=w520:u32)
    n261 = To Unsigned Long Integer(number=w515) -> (unsigned 32bit integer=w519:u32)
    n262 = xnode "Read/Write Control"("FPGA VI Reference In"=w541, "error in"=w539, "ton"=w538, "tof"=w530, "ton 2"=w537, "tof 2"=w529, "ton 3"=w536, "tof 3"=w528, "ton 4"=w535, "tof 4"=w527, "ton 5"=w526, "tof 5"=w525, "ton 6"=w524, "tof 6"=w523, "ton 7"=w522, "tof 7"=w521, "ton 8"=w520, "tof 8"=w519, "E1O"=w514, "E2O"=w514, "E3O"=w514, "E4O"=w514, "E5O"=w514, "E6O"=w514, "E7O"=w514, "E8O"=w514, "EI1"=w513, "EI2"=w513, "EI3"=w513, "EI4"=w513, "EI54"=w513, "EI6"=w513, "EI7"=w513, "EI8"=w513, "En1"=w491, "En2"=w490, "En3"=w489, "En4"=w488, "En5"=w512, "En6"=w511, "En7"=w510, "En8"=w509) -> ("FPGA VI Reference Out"=w542:refnum<k20>, "error out"=w540:errorcluster)
    n263 = local read "STOP Indicator"() -> (w553:bool)
  }
  n264 = timed-loop {
    timing: w43 -> [_]
    timing-out: [_] -> w42
    tunnel: [w616] -> w41
    tunnel: [w615] -> w40
    tunnel: w31 -> [w614]
    tunnel: w30 -> [w613]
    stop <- w619 stop-if-true
    w598 = u32 250 ("Trigger pulse interval 1")
    # "Ultrasonic Sensor"
    n265 = node-c288() -> ()  [unwired: 1 in, 1 out]
    n266 = xnode "Invoke Method"("FPGA VI Reference In"=w614, "error in"=w613) -> ("FPGA VI Reference Out"=w612:refnum<k20>, "error out"=w611:errorcluster)  [unwired: 1 in]
    n267 = call <vilib>:"FL Load Fuzzy System.vi"("file path"=path "c:/obstacle MOM.fs") -> ("error out"=w600:errorcluster, "fuzzy system out"=w601:T8)  [unwired: 1 in, 8 out]
    n268 = xnode "Read/Write Control"("FPGA VI Reference In"=w612, "error in"=w611, "Trigger pulse interval 1"=w598, "Trigger pulse interva 2"=w598, "Trigger pulse interval 3"=w598, "Trigger pulse interval 4"=w598) -> ("FPGA VI Reference Out"=w618:refnum<k20>, "error out"=w617:errorcluster)
    n269 = xnode "Read/Write Control"("FPGA VI Reference In"=w618, "error in"=w617) -> ("FPGA VI Reference Out"=w616:refnum<k20>, "error out"=w615:errorcluster, "time of flight 1"=w610:u32, "time of flight 2"=w609:u32, "time of flight 3"=w606:u32, "time of flight 4"=w604:u32)
    "US1" <- w610
    "US2" <- w609
    "US3" <- w606
    "US 4" <- w604
    n270 = Multiply(x=w604, y=sgl 0.016967773) -> (x*y=w596:sgl)
    "ultrasonik4" <- w596
    n271 = Multiply(x=w606, y=sgl 0.016967773) -> (x*y=w595:sgl)
    "ultrasonik3" <- w595
    n272 = Multiply(x=w610, y=sgl 0.016967773) -> (x*y=w594:sgl)
    "ultrasonik1" <- w594
    n273 = Multiply(x=w609, y=sgl 0.016967773) -> (x*y=w593:sgl)
    "ultrasonik2" <- w593
    n274 = Build Array(w594, w593, w595, w596) -> (w603:sgl[])
    n275 = call-poly <vilib>:"FL Fuzzy Controller.vi"("error in (no error)"=w600, "input values"=w603, "fuzzy system in"=w601) -> ("output values"=w602:dbl[])  [unwired: 8 out]
    n276 = Index Array(array=w602) -> (element #1=→"kecp.kiri":dbl, element #2=→"kecp.kanan":dbl, element #3=→"var.auto":dbl)  [unwired: 3 in]
    n277 = local read "STOP Indicator"() -> (w619:bool)
    n278 = node-c288() -> ()  [unwired: 1 in, 1 out]
  }
  n279 = node-c288(w34) -> ()  [unwired: 1 out]
  n280 = xnode "Close FPGA VI Reference"("FPGA VI Reference In"=w33, "error in"=w32) -> ()  [unwired: 1 out]
  n281 = node-c288(w42) -> ()  [unwired: 1 out]
  n282 = xnode "Close FPGA VI Reference"("FPGA VI Reference In"=w41, "error in"=w40) -> ()  [unwired: 1 out]
  n283 = node-c288(w38) -> ()  [unwired: 1 out]
  n284 = xnode "Close FPGA VI Reference"("FPGA VI Reference In"=w37, "error in"=w36) -> ()  [unwired: 1 out]
  n285 = xnode "Close FPGA VI Reference"("FPGA VI Reference In"=w45, "error in"=w44) -> ()  [unwired: 1 out]
